vi "GPIO_Control.vi"(0 "Device address":i32=4660 format="%x") -> ()   [LabVIEW 2011]
doc: "This VI is a pop-up window that allows full access to the control, and measure bits. This should be included with all USB-DAQ / DIG applications as a debug tool. You can also look through the software as an example of how to configure the control and measure bits."
panel:
  out "result":u16 format="%x"
  in  "Read Meas Bits":bool
  in  "Set Control Bits":bool
  out "MES8":u16
  out "MES7":u16
  out "MES6":u16
  out "MES5":u16
  out "MES4":u16
  out "MES3":u16
  out "MES2":u16
  out "MES1":u16
  in  "CTR1":u16 max=1
  in  "CTR2":u16 max=1
  in  "CTR3":u16 max=1
  in  "CTR4":u16 max=1
  in  "CTR5":u16 max=1
  in  "CTR6":u16 max=1
  in  "CTRL7":u16 max=1
  in  "CTRL8":u16 max=1
  # "for internal use only \ndon't include in user interface"
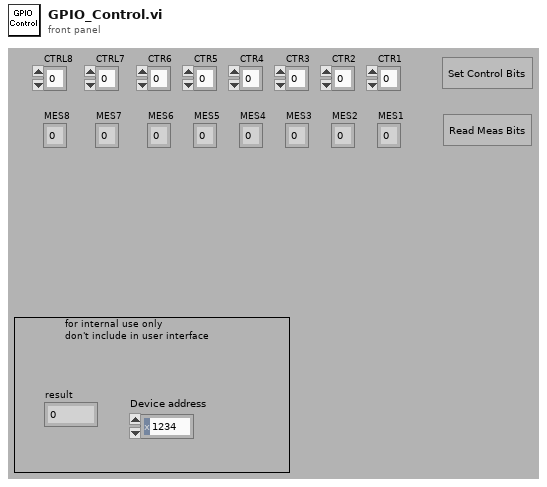
[diagram p1: front panel]
types:
  T1 = enum32{"Invalid", "Standard", "Closed", "Hidden", "Minimized", "Maximized"}
  T2 = enum16{"Always On", "Always Off", "Off While Running"}
  T3 = enum32{"invalid app kind", "Development System", "Run Time System", "Student Edition", "Embedded LabVIEW", "Evaluation", "Custom"}
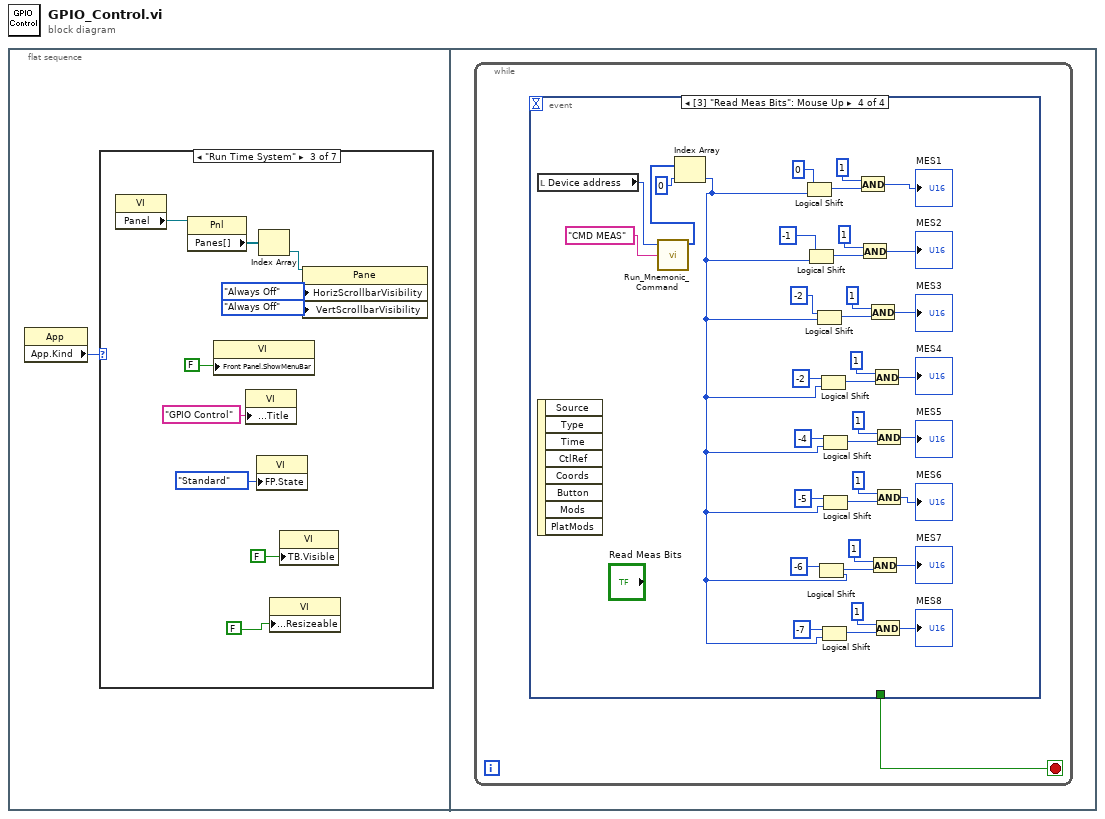
[diagram p0: block diagram]
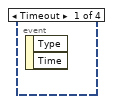
[diagram p8: hidden frame]
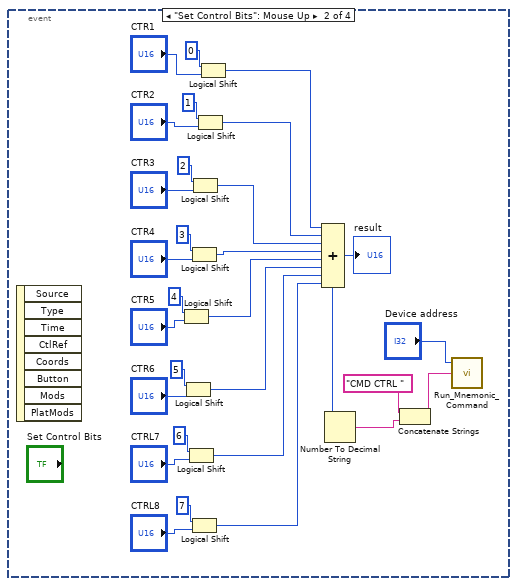
[diagram p9: hidden frame]
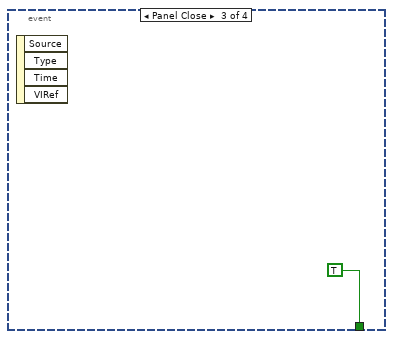
[diagram p10: hidden frame]
diagram:
  n1 = flat-sequence {
    frame #0 {
      n2 = property class="App"() -> ("App.Kind"=w1:T3)  [unwired: 2 in, 2 out]
      n3 = case shown="\"Run Time System\"" w1 {
        frame "invalid app kind", Default {
        }
        frame "Development System" {
        }
        frame "Run Time System" {
          n4 = property class="VI"() -> ("Panel"=w11:refnum<vi>)  [unwired: 2 in, 2 out]
          n5 = property class="Pnl"(reference=w11) -> ("Panes[]"=w10:refnum<vi>[])  [unwired: 1 in, 2 out]
          n6 = property class="VI"("Front Panel.ShowMenuBar"=FALSE ("Front Panel Window:Show Menu Bar")) -> ()  [unwired: 2 in, 2 out]
          n7 = property class="VI"("Front Panel.Title"="GPIO Control" ("Front Panel Window:Title")) -> ()  [unwired: 2 in, 2 out]
          n8 = property class="VI"("FP.State"=T1."Standard" ("Front Panel Window:State")) -> ()  [unwired: 2 in, 2 out]
          n9 = Index Array(array=w10) -> (element=w9:refnum<vi>)  [unwired: 1 in]
          n10 = property class="VI"("Front Panel.Resizeable"=FALSE ("Front Panel Window:Resizeable")) -> ()  [unwired: 2 in, 2 out]
          n11 = property class="VI"("TB.Visible"=FALSE ("Front Panel Window:Resizeable")) -> ()  [unwired: 2 in, 2 out]
          n12 = property class="Pane"(reference=w9, "HorizScrollbarVisibility"=T2."Always Off" ("Horizontal Scrollbar Visibility"), "VertScrollbarVisibility"=T2."Always Off" ("Vertical Scrollbar Visibility")) -> ()  [unwired: 1 in, 2 out]
        }
        frame "Student Edition" {
        }
        frame "Embedded LabVIEW" {
        }
        frame "Evaluation" {
        }
        frame "Custom" {
        }
      }
    }
    frame #1 {
      n13 = while {
        stop <- w12 stop-if-true
        n14 = event shown="[3] \"Read Meas Bits\": Mouse Up" {
          selector: _ -> [_ _ _ _]
          dyn-events: _ -> [_ _ _ _]
          timeout: _ -> [_ _ _ _]
          tunnel: [_ _ TRUE _] -> w12
          event Timeout {
            n15 = event-data() -> ()  [unwired: 1 in, 2 out]
          }
          event "Set Control Bits": Mouse Up {
            n16 = event-data() -> ()  [unwired: 1 in, 8 out]
            n17 = Logical Shift(y=i16 4, x="CTR5") -> (x << y=w21:u16)
            n18 = Logical Shift(y=i16 5, x="CTR6") -> (x << y=w20:u16)
            n19 = Logical Shift(y=i16 6, x="CTRL7") -> (x << y=w19:u16)
            n20 = Logical Shift(y=i16 3, x="CTR4") -> (x << y=w22:u16)
            n21 = Logical Shift(y=i16 7, x="CTRL8") -> (x << y=w18:u16)
            n22 = Logical Shift(y=i16 2, x="CTR3") -> (x << y=w23:u16)
            n23 = Logical Shift(y=i16 1, x="CTR2") -> (x << y=w24:u16)
            n24 = Logical Shift(y=i16 0, x="CTR1") -> (x << y=w25:u16)
            n25 = Compound Arithmetic op=ADD(w25, w24, w23, w22, w21, w20, w19, w18) -> (w17:u16)
            "result" <- w17
            n26 = Number To Decimal String(number=w17) -> (decimal integer string=w15:string)  [unwired: 1 in]
            n27 = Concatenate Strings("CMD CTRL " ("string"), w15) -> (w13:string)
            n28 = call "Run_Mnemonic_Command.vi"("command string"=w13, "Device address"="Device address") -> ()  [unwired: 2 in, 5 out]
          }
          event Panel Close {
            n29 = event-data() -> ()  [unwired: 1 in, 4 out]
          }
          event "Read Meas Bits": Mouse Up {
            n30 = local read "Device address"() -> (w45:i32)
            n31 = event-data() -> ()  [unwired: 1 in, 8 out]
            n32 = call "Run_Mnemonic_Command.vi"("command string"="CMD MEAS", "Device address"=w45) -> ("result-array"=w43:u8[])  [unwired: 2 in, 4 out]
            n33 = Index Array(array=w43, index=0) -> (element=w46:u8)
            n34 = Logical Shift(y=i16 0, x=w46) -> (x << y=w78:u8)
            n35 = Logical Shift(y=i16 -1, x=w46) -> (x << y=w75:u8)
            n36 = Logical Shift(y=i16 -2, x=w46) -> (x << y=w71:u8)
            n37 = Logical Shift(y=i16 -6, x=w46) -> (x << y=w55:u8)
            n38 = Logical Shift(y=i16 -2, x=w46) -> (x << y=w67:u8)
            n39 = Logical Shift(y=i16 -7, x=w46) -> (x << y=w52:u8)
            n40 = Logical Shift(y=i16 -4, x=w46) -> (x << y=w63:u8)
            n41 = Logical Shift(y=i16 -5, x=w46) -> (x << y=w59:u8)
            n42 = And(x=i16 1, y=w78) -> (x .and. y?=→"MES1":i16)
            n43 = And(x=i16 1, y=w75) -> (x .and. y?=→"MES2":i16)
            n44 = And(x=i16 1, y=w71) -> (x .and. y?=→"MES3":i16)
            n45 = And(x=i16 1, y=w55) -> (x .and. y?=→"MES7":i16)
            n46 = And(x=i16 1, y=w67) -> (x .and. y?=→"MES4":i16)
            n47 = And(x=i16 1, y=w52) -> (x .and. y?=→"MES8":i16)
            n48 = And(x=i16 1, y=w63) -> (x .and. y?=→"MES5":i16)
            n49 = And(x=i16 1, y=w59) -> (x .and. y?=→"MES6":i16)
          }
        }
      }
    }
  }
